vi "ConvertCameraSettings.vi"(1 "Saved Settings:":T2={"Requested Genlock "="20140911165611", "Min Frame Clocks "="20140911165611", "Is Seq Clk Freq "="20140911165611", "Pretrigger Frames "="20140911165611", "Duration "="20140911165611", "Overclock "="20140911165611", "Requested Horizontal "="20140911165611", "Frames "="20140911165611", "Requested Pretrigger "="20140911165611", "Words per Frame "="20140911165611", "Buffer End "="20140911165611", "Clocks per Frame  "="20140911165611", "Requested Duration "="20140911165611", "Pretrigger "="20140911165611", "Post-trigger Frames "="20140911165611", "Vertical "="20140911165611", "Requested Vertical "="20140911165611", "Reqested Frame Rate "="20140911165611", "Frame Rate "="20140911165611", "Horizontal "="20140911165611", "Clocks per Exposure "="20140911165611", "Digital Gain "="20140911165611", "Exposure "="20140911165611", "Genlock "="20140911165611", "Analog Gain "="20140911165611", "Subsample "="20140911165611", "Requested Exposure "="20140911165611", "Iso "="20140911165611", "Requested Overclock "="20140911165611", "Requested Subsample "="20140911165611", "Requested Iso"="20140911165611", "Multishot"="20140911165611", "Requested Multishot"="20140911165611", "Monochrome"="20140911165611", "Requested mono"="20140911165611", "FPGA Temp"="20140911165611", "Is Temp"="20140911165611", "Posttrigger Duration"="20140911165611", "Pretrigger Duration"="20140911165611", "dacvrefadc"="20140911165611"}) -> (0 "Settings":T1={"Frame Rate (fps)"=1000.0, "Exposure (1/sec)"=1500.0, "Horizonal"=0, "Vertical"=0, "ISO"=500, "Duration"=1.0, "Pretrigger (%)"=50.0, "MultiShot"=1, "Subsample?"=FALSE, "Force Mono?"=FALSE, "Genlock"=enum."Off", "Overclock"=enum."Off"} {"Pretrigger (%)" min=0.0 max=100.0 step=1.0; "ISO" min=0 max=1600 step=1; "Exposure (1/sec)" min=4e-06 max=250000.0 step=1.0; "Frame Rate (fps)" min=0.1 max=25000.0 step=1.0})   [LabVIEW 2015]
uses:
  SettingsCtrl.ctl
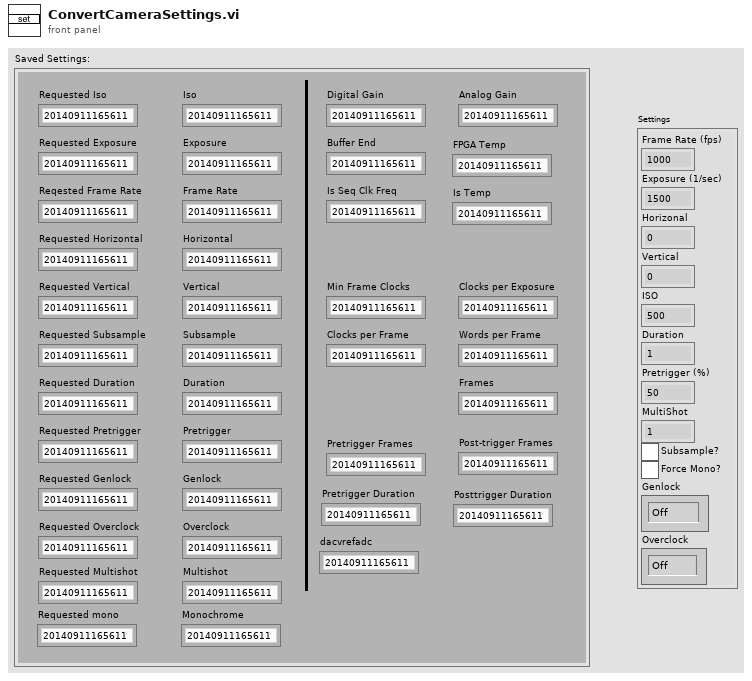
[diagram p1: front panel]
types:
  T1 = cluster{"Frame Rate (fps)":dbl, "Exposure (1/sec)":dbl, "Horizonal":u16, "Vertical":u16, "ISO":i16, "Duration":dbl, "Pretrigger (%)":dbl, "MultiShot":i16, "Subsample?":bool, "Force Mono?":bool, "Genlock":enum16{"Off", "Master", "Slave"}, "Overclock":enum16{"Off", "A level", "B Level", "C Level", "D Level"}}
  T2 = typedef "SettingsCtrl.ctl" = cluster{"Requested Genlock ":string, "Min Frame Clocks ":string, "Is Seq Clk Freq ":string, "Pretrigger Frames ":string, "Duration ":string, "Overclock ":string, "Requested Horizontal ":string, "Frames ":string, "Requested Pretrigger ":string, "Words per Frame ":string, "Buffer End ":string, "Clocks per Frame  ":string, "Requested Duration ":string, "Pretrigger ":string, "Post-trigger Frames ":string, "Vertical ":string, "Requested Vertical ":string, "Reqested Frame Rate ":string, "Frame Rate ":string, "Horizontal ":string, "Clocks per Exposure ":string, "Digital Gain ":string, "Exposure ":string, "Genlock ":string, "Analog Gain ":string, "Subsample ":string, "Requested Exposure ":string, "Iso ":string, "Requested Overclock ":string, "Requested Subsample ":string, "Requested Iso":string, "Multishot":string, "Requested Multishot":string, "Monochrome":string, "Requested mono":string, "FPGA Temp":string, "Is Temp":string, "Posttrigger Duration":string, "Pretrigger Duration":string, "dacvrefadc":string}
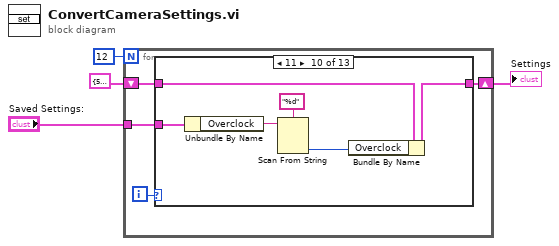
[diagram p0: block diagram]
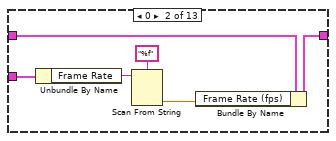
[diagram p3: hidden frame]
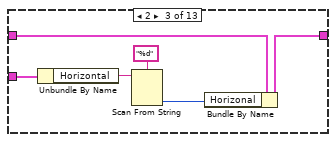
[diagram p4: hidden frame]
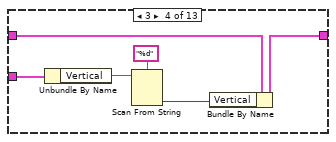
[diagram p5: hidden frame]
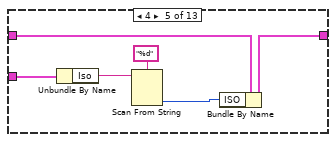
[diagram p6: hidden frame]
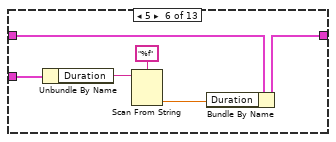
[diagram p7: hidden frame]
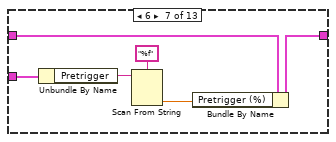
[diagram p8: hidden frame]
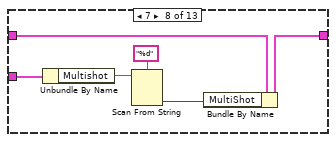
[diagram p9: hidden frame]
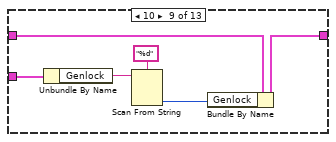
[diagram p10: hidden frame]
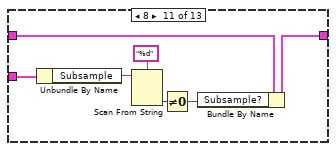
[diagram p11: hidden frame]
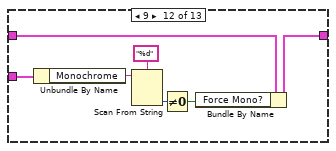
[diagram p12: hidden frame]
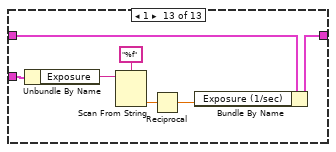
[diagram p13: hidden frame]
diagram:
  n1 = for {
    N: 12 -> [_]
    tunnel: "Saved Settings:" -> [w8]
    shift-right: [w5] -> w1
    shift-left: T1 {"Frame Rate (fps)"=5740.817777777779, "Exposure (1/sec)"=6053.590834728392, "Horizonal"=1280, "Vertical"=294, "ISO"=500, "Duration"=1.0, "Pretrigger (%)"=50.0, "MultiShot"=1, "Subsample?"=FALSE, "Force Mono?"=FALSE, "Genlock"=enum."Off", "Overclock"=enum."Off"} ("Settings") -> [w6]
    i -> [w7]
    n2 = case shown="11" w7 {
      tunnel: w8 -> [_ w15 w21 w27 w33 w39 w45 w51 w57 w63 w70 w77 w84]
      tunnel: w6 -> [w9 w11 w17 w23 w29 w35 w41 w47 w53 w59 w66 w73 w80]
      tunnel: [w9 w10 w16 w22 w28 w34 w40 w46 w52 w58 w65 w72 w79] -> w5
      frame Default {
      }
      frame 0 {
        n3 = Unbundle By Name(w15) -> ("Frame Rate"=w14:string)
        n4 = Scan From String(format string="%f", input string=w14) -> (output 1=w12:dbl)  [unwired: 3 in, 3 out]
        n5 = Bundle By Name(cluster=w11, "Frame Rate (fps)"=w12) -> (w10:T1)
      }
      frame 2 {
        n6 = Unbundle By Name(w21) -> ("Horizontal"=w20:string)
        n7 = Scan From String(format string="%d", input string=w20) -> (output 1=w18:i32)  [unwired: 3 in, 3 out]
        n8 = Bundle By Name(cluster=w17, "Horizonal"=w18) -> (w16:T1)
      }
      frame 3 {
        n9 = Unbundle By Name(w27) -> ("Vertical"=w26:string)
        n10 = Scan From String(format string="%d", input string=w26) -> (output 1=w24:i32)  [unwired: 3 in, 3 out]
        n11 = Bundle By Name(cluster=w23, "Vertical"=w24) -> (w22:T1)
      }
      frame 4 {
        n12 = Unbundle By Name(w33) -> ("Iso"=w32:string)
        n13 = Scan From String(format string="%d", input string=w32) -> (output 1=w30:i32)  [unwired: 3 in, 3 out]
        n14 = Bundle By Name(cluster=w29, "ISO"=w30) -> (w28:T1)
      }
      frame 5 {
        n15 = Unbundle By Name(w39) -> ("Duration"=w38:string)
        n16 = Scan From String(format string="%f", input string=w38) -> (output 1=w36:dbl)  [unwired: 3 in, 3 out]
        n17 = Bundle By Name(cluster=w35, "Duration"=w36) -> (w34:T1)
      }
      frame 6 {
        n18 = Unbundle By Name(w45) -> ("Pretrigger"=w44:string)
        n19 = Scan From String(format string="%f", input string=w44) -> (output 1=w42:dbl)  [unwired: 3 in, 3 out]
        n20 = Bundle By Name(cluster=w41, "Pretrigger (%)"=w42) -> (w40:T1)
      }
      frame 7 {
        n21 = Unbundle By Name(w51) -> ("Multishot"=w50:string)
        n22 = Scan From String(format string="%d", input string=w50) -> (output 1=w48:i32)  [unwired: 3 in, 3 out]
        n23 = Bundle By Name(cluster=w47, "MultiShot"=w48) -> (w46:T1)
      }
      frame 10 {
        n24 = Unbundle By Name(w57) -> ("Genlock"=w56:string)
        n25 = Scan From String(format string="%d", input string=w56) -> (output 1=w54:i32)  [unwired: 3 in, 3 out]
        n26 = Bundle By Name(cluster=w53, "Genlock"=w54) -> (w52:T1)
      }
      frame 11 {
        n27 = Unbundle By Name(w63) -> ("Overclock"=w62:string)
        n28 = Scan From String(format string="%d", input string=w62) -> (output 1=w60:i32)  [unwired: 3 in, 3 out]
        n29 = Bundle By Name(cluster=w59, "Overclock"=w60) -> (w58:T1)
      }
      frame 8 {
        n30 = Unbundle By Name(w70) -> ("Subsample"=w69:string)
        n31 = Scan From String(format string="%d", input string=w69) -> (output 1=w67:i32)  [unwired: 3 in, 3 out]
        n32 = Not Equal To 0?(x=w67) -> (x != 0?=w64:bool)
        n33 = Bundle By Name(cluster=w66, "Subsample?"=w64) -> (w65:T1)
      }
      frame 9 {
        n34 = Unbundle By Name(w77) -> ("Monochrome"=w76:string)
        n35 = Scan From String(format string="%d", input string=w76) -> (output 1=w74:i32)  [unwired: 3 in, 3 out]
        n36 = Not Equal To 0?(x=w74) -> (x != 0?=w71:bool)
        n37 = Bundle By Name(cluster=w73, "Force Mono?"=w71) -> (w72:T1)
      }
      frame 1 {
        n38 = Unbundle By Name(w84) -> ("Exposure"=w83:string)
        n39 = Scan From String(format string="%f", input string=w83) -> (output 1=w81:dbl)  [unwired: 3 in, 3 out]
        n40 = Reciprocal(x=w81) -> (1/x=w78:dbl)
        n41 = Bundle By Name(cluster=w80, "Exposure (1/sec)"=w78) -> (w79:T1)
      }
    }
  }
  "Settings" <- w1
